vi "Affinities.vi"   [LabVIEW 2020]
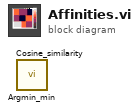
[diagram p0: block diagram]
diagram:
  n1 = call "Argmin_min.vi"() -> ()  [unwired: 10 in, 2 out]
  n2 = call "Cosine_similarity.vi"() -> ()  [unwired: 10 in, 2 out]
